vi "Main FPGA 8-axis with Limits and changes 16DIO.vi"() -> ()   [LabVIEW 2013]
uses:
  <vilib>/Motion/MotorControl/_s/nism.interpretControlRegister.stateTransition.ctl
  <vilib>/Platform/TimedLoop/XDataNode/timing_clust.ctl
  <vilib>/Platform/TimedLoop/XDataNode/nitl_modes.ctl
  <vilib>/Platform/TimedLoop/XDataNode/wakeup.ctl
  <vilib>/rvi/Emulation/niFpgaSctlEmulationGetInTimedLoop.vi
  <vilib>/rvi/Emulation/niFpgaEmulationReportErrorSimple.vi
  <vilib>/rvi/Emulation/niFpgaGetClockAttributes.vi
  <vilib>/rvi/Emulation/niFpgaCriticalErrorInLSC.vi
  Global FPGA 8-axis.vi
  <vilib>/rvi/eio/common/nirviEmuTemplateMethod_errors.vi
  <vilib>/Motion/SoftMotion/Synchronization/nism.rioScan.generateSyncScan.vi
  <vilib>/rvi/Emulation/niFpgaProcessEmulError.vi
  <vilib>/Motion/MotorControl/_s/nism.interpretControlRegister.indexed.vi
  <vilib>/Motion/MotorControl/_s/nism.generateStatusRegister.indexed.vi
  <vilib>/Motion/MotorControl/_s/nism.mdo.read.dio.portA.2.vi
  <vilib>/Motion/MotorControl/_s/nism.mdo.read.positionLoopSyncData.vi
  <vilib>/Motion/MotorControl/_s/nism.mdo.read.splineData.vi
  <vilib>/Motion/MotorControl/_s/nism.splineInterpolation.fxp.3.index.vi
  <vilib>/Motion/MotorControl/_s/nism.mdo.handler.indexed.vi
  <vilib>/Platform/TimedLoop/XDataNode/XDataNode.xnode
  <vilib>/eio/EIONode/EIONode.xnode
  <vilib>/Motion/MotorControl/NI_SoftMotion_MotorControlIP.lvlib
  <vilib>/Platform/TimedLoop/XDataNode/XDNodeRunTimeDep.lvlib
  <vilib>/Motion/SoftMotion/Synchronization/NI_SoftMotion_Synchronization.lvlib
panel:
  out "DI (8bits)":u8
  in  "DO (8bits)":u32
  out "Axis Positions":fxp<+/-,64,32>[](array[numeric])
  in  "STEP or CW? (T=STEP)":bool
  out "Drive Enable":bool[](array[boolean])
  in  "Enable Watchdog":bool
  in  "Pet Watchdog":bool
  in  "Watchdog Timeout Period (ticks)":u64=40000000 format="%.0p"
  out "Watchdog Timed Out?":bool
  out "Time Since Last Pet":u64
  in  "Enable value":bool
  in  "Drive Enable override?":bool
  out "State":T1=enum."Start --> Initializing" caption="state transition"
  in  "Sync Value":bool
  in  "Sync Enable override?":bool
  in  "Invert direction?":bool
  out "Sync is Fault":bool
  out "Sync is Locked":bool
  in  "minimum pulse":u16=40
  # "Synchronization Loop"
  # "Control Status Loop"
  # "Notes: \n1. This VI provides the communication interface between the NI SoftMotion Engine and the LabVIEW FPGA Module. You must compile this VI for a specific FPGA target before use. After compiling, run the VI before running any of the Express VI examples. For information on moving this example to another FPGA target, refer to ni.com/info and enter info code fpgaex.\n\n2. Only use the Reset Axis button if you are unable to communicate with the axis by any other means. This button resets the device state machine and other VIs to a known state. After resetting the axis, switch the NI Scan Engine from Active Mode to Configuration Mode, then back to Active Mode, before attempting to enable the axis."
  # "(These two buttons \nare for testing\npurposes.)"
  # "(These two buttons \nare for testing\npurposes.)"
  # "Step/Direction Loop"
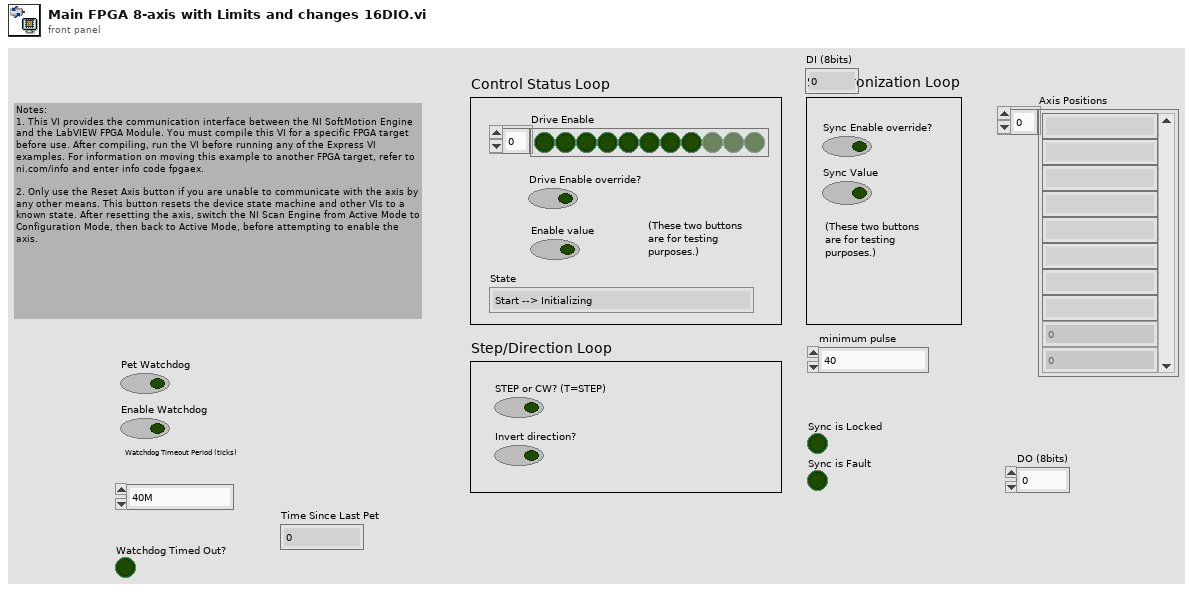
[diagram p1: front panel]
types:
  T1 = typedef "NI_SoftMotion_MotorControlIP.lvlib/nism.interpretControlRegister.stateTransition.ctl" = enum8{"Invalid", "Start --> Initializing", "Initializing --> Disabled", "Disabled --> Ready To Switch On", "Ready To Switch On --> Switched On", "Ready To Switch On --> Disable", "Switched On --> Operation Enable", "Switched On --> Ready To Switch On", "Switched On --> Disabled", "Operation Enable --> Switched On", "Operation Enable --> Ready To Switch On", "Operation Enable --> Disabled", "Fault --> Disabled", "Any --> Fault", "None"}
  T2 = typedef "NI_SoftMotion_MotorControlIP.lvlib/nism.dio.portA.config.2.ctl" = cluster{"digital filter (us)":u16[], "safe state":enum16{"Low", "High", "No Change"}[]}
  T3 = typedef "NI_SoftMotion_MotorControlIP.lvlib/nism.mdo.splineData.ctl" = cluster{"spline type":T4, "traj per/spline per":u16, "spline per/traj per":fxp<+,32,0>}
  T4 = typedef "nism.splineInterpolation.type.ctl" = u16
  T5 = typedef "NI_SoftMotion_Synchronization.lvlib/nism.softmotionScan.timerConfig.ctl" = cluster{"Target Period (clocks)":u16, "Host Period / Target Period":u16}
  T6 = typedef "NI_SoftMotion_Synchronization.lvlib/nism.softmotionScan.timerControl.ctl" = cluster{"SM Scan":bool, "SM Scan Count":u32, "SM Scan Enabled":bool}
  T7 = typedef "XDNodeRunTimeDep.lvlib/timing_clust.ctl" = cluster{"Expected End [f-1]":u64, "Actual End [f-1]":u64, "Finished Late? [f-1]":bool, "Expected End [i-1]":u64, "Actual End [i-1]":u64, "Finished Late? [i-1]":bool, "Expected Start [i]":u64, "Actual Start [i]":u64, "Expected Start [f]":u64, "Actual Start [f]":u64, "Source Name":string, "Structure Name":string, "Period":i64, "Deadline":i64, "Offset":i64, "Start":i64, "Priority":i32, "Timeout":i32, "Mode":T8, "Wakeup Reason":T9, "Error":errorcluster, "Source Type":string, "Secondary Source Type":string, "Global End Time":u64, "Global Start Time":u64, "Frame Duration":u64, "Iteration Duration":u64, "Assigned CPU":i32, "I/O Scan Engine Mode":u32}
  T8 = typedef "XDNodeRunTimeDep.lvlib/nitl_modes.ctl" = enum32{"No Change", "Process missed periods, maintain original phase", "Discard missed periods, maintain original phase", "Process missed periods, ignore original phase", "Discard missed periods, ignore original phase"}
  T9 = typedef "XDNodeRunTimeDep.lvlib/wakeup.ctl" = enum32{"Normal", "Aborted", "Asynchronous wakeup", "Timing source error", "Timed loop error", "Timeout"}
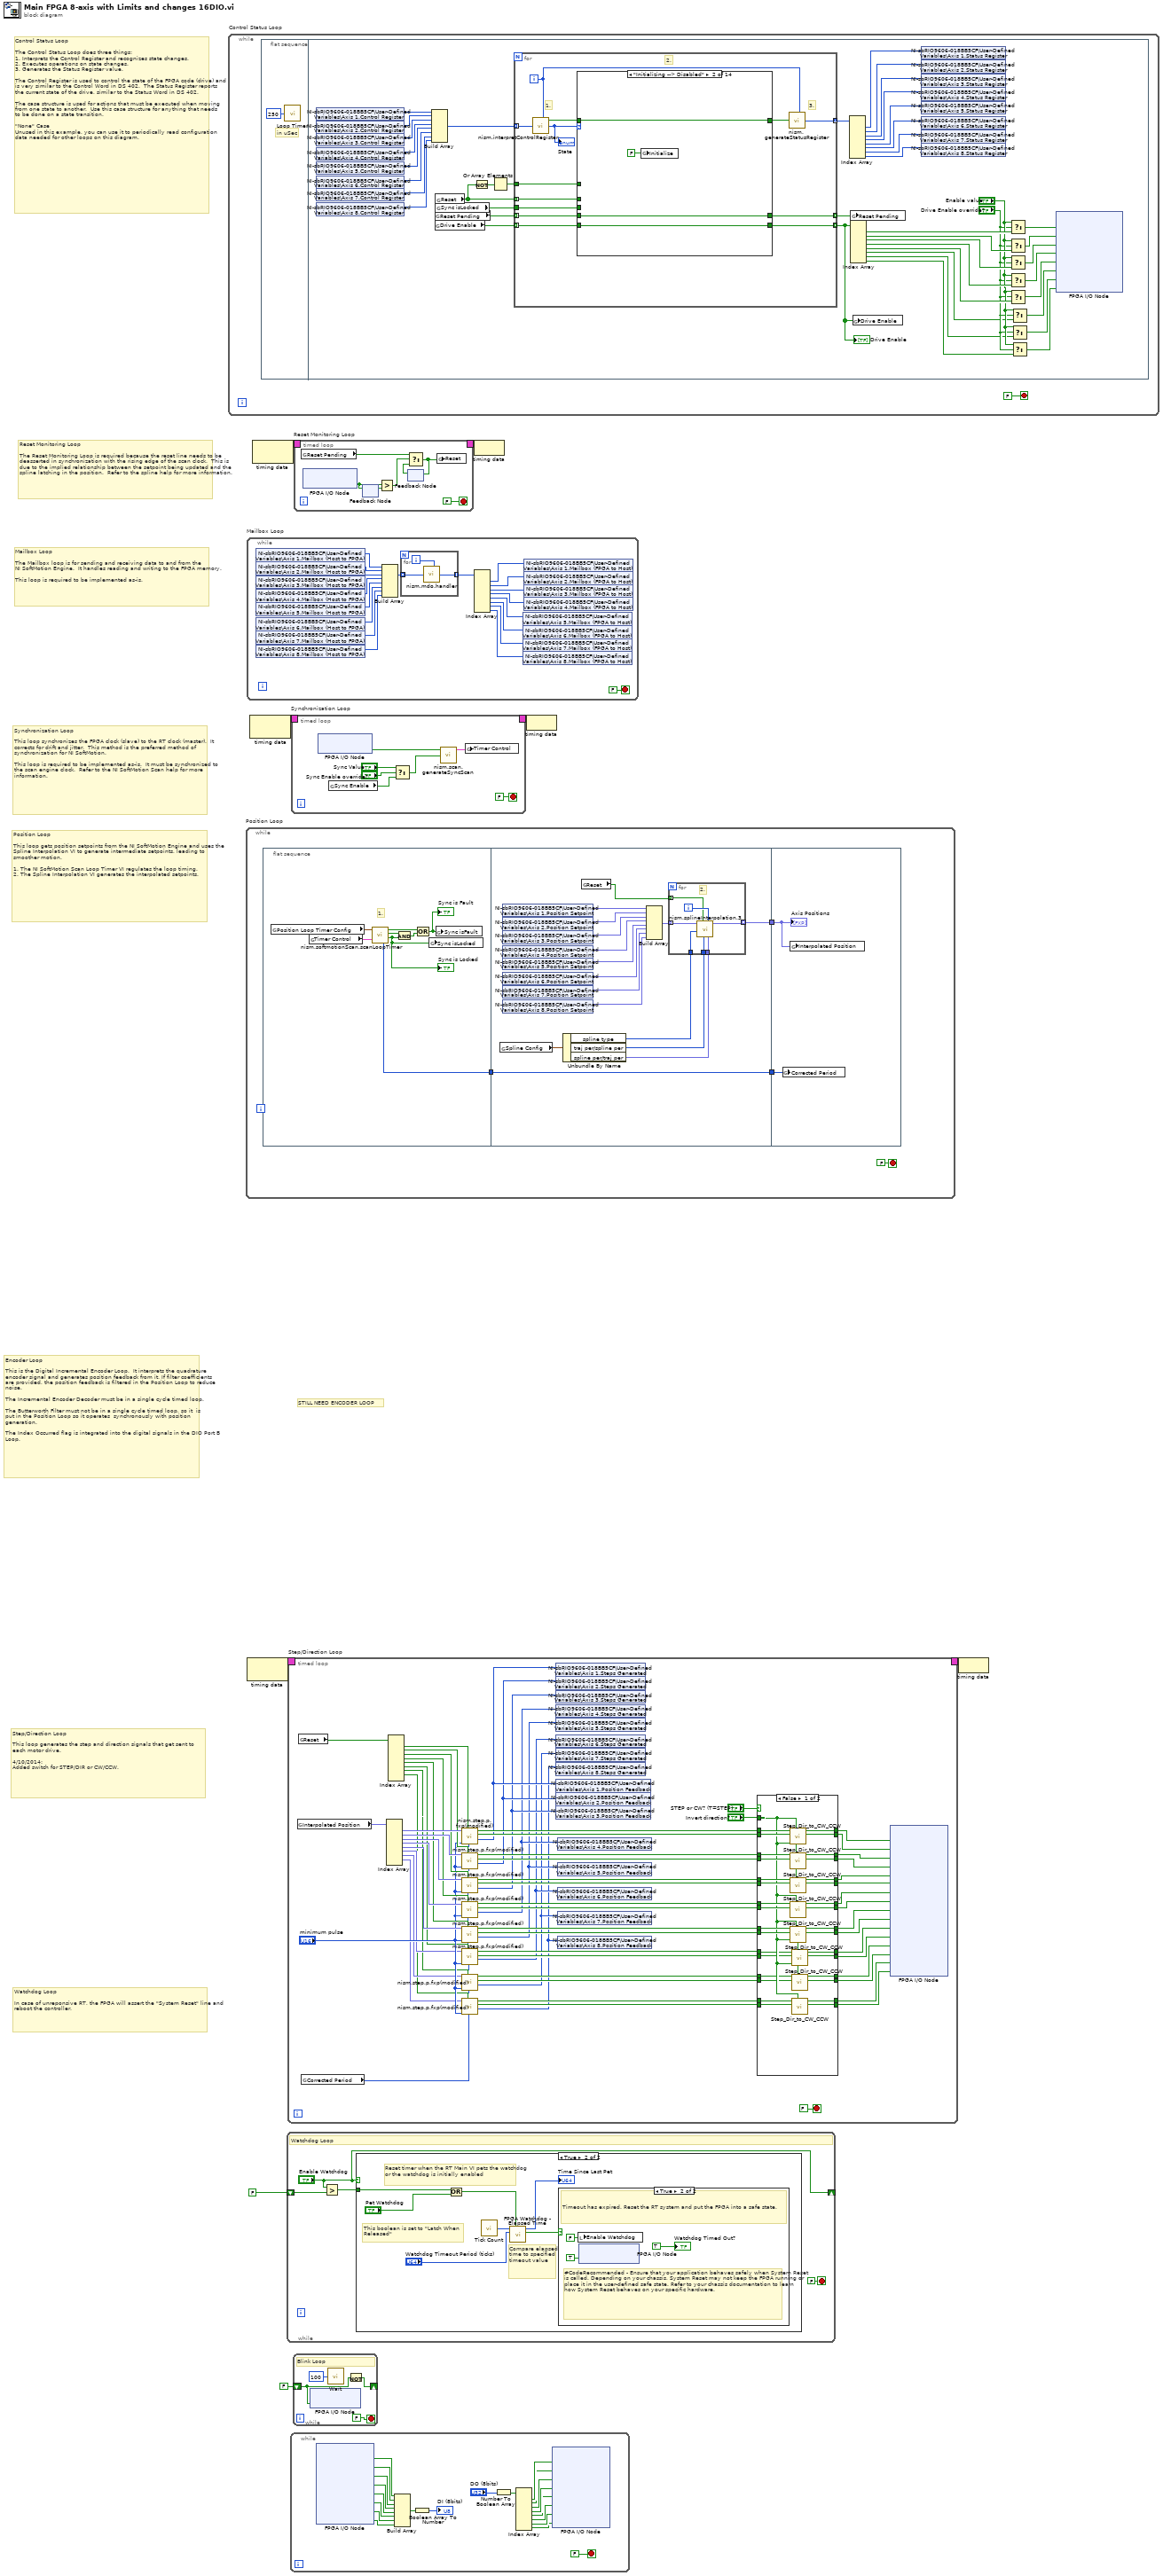
[diagram p0: block diagram]
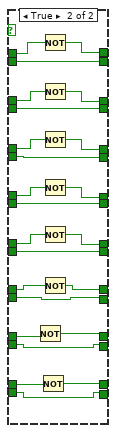
[diagram p5: hidden frame]
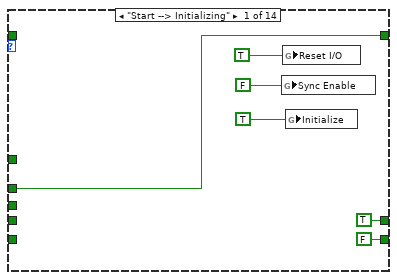
[diagram p6: hidden frame]
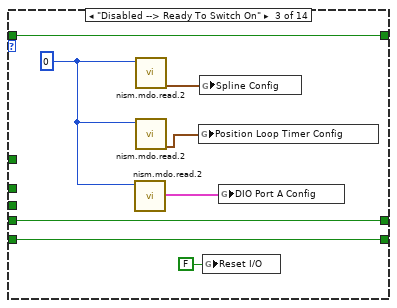
[diagram p7: hidden frame]
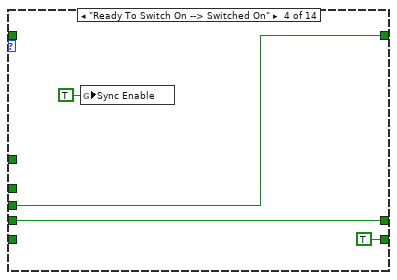
[diagram p8: hidden frame]
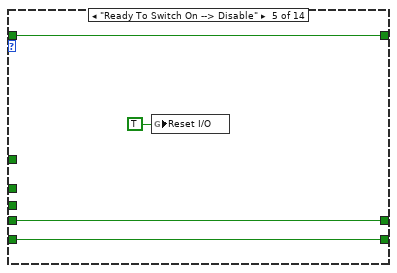
[diagram p9: hidden frame]
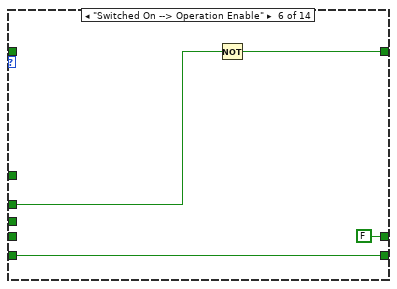
[diagram p10: hidden frame]
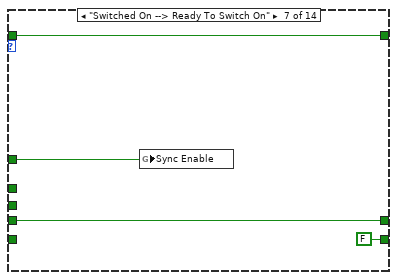
[diagram p11: hidden frame]
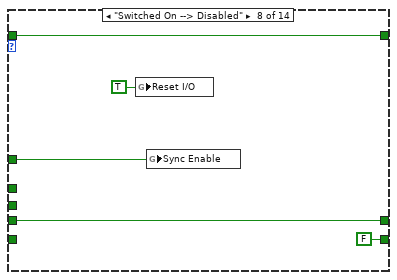
[diagram p12: hidden frame]
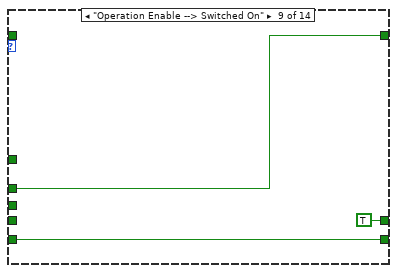
[diagram p13: hidden frame]
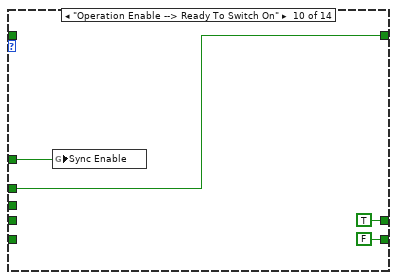
[diagram p14: hidden frame]
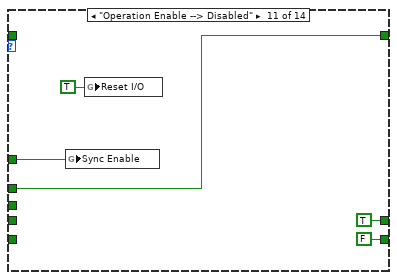
[diagram p15: hidden frame]
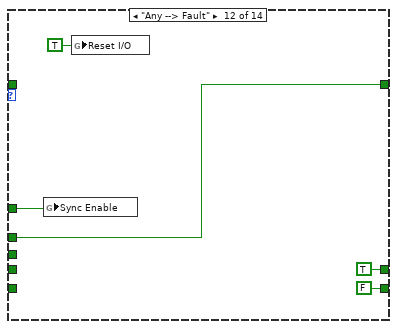
[diagram p16: hidden frame]
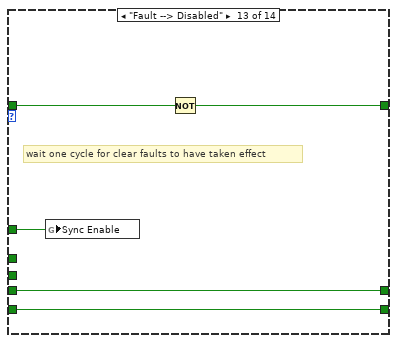
[diagram p17: hidden frame]
diagram:
  # "STILL NEED ENCODER LOOP"
  # "Encoder Loop\n\nThis is the Digital Incremental Encoder Loop.  It interprets the quadrature encoder signal and generates position feedback from it. If filter coefficients are provided, the position feedback is filtered in the Position Loop to reduce noise.\n\nThe Incremental Encoder Decoder must be in a single cycle timed loop.\n\nThe Butterworth Filter must not be in a single cycle timed loop, so it  is\nput in the Position Loop so it operates  synchronously with position generation.\n\nThe Index Occurred flag is integrated into the digital signals in the DIO Port B Loop."
  # "Watchdog Loop\n\nIn case of unreponsive RT, the FPGA will assert the \"System Reset\" line and reboot the controller."
  # "Step/Direction Loop\n\nThis loop generates the step and direction signals that get sent to \neach motor drive.\n\n4/10/2014:\nAdded switch for STEP/DIR or CW/CCW."
  # "Position Loop\n\nThis loop gets position setpoints from the NI SoftMotion Engine and uses the Spline Interpolation VI to generate intermediate setpoints, leading to smoother motion.\n\n1. The NI SoftMotion Scan Loop Timer VI regulates the loop timing. \n2. The Spline Interpolation VI generates the interpolated setpoints."
  # "Synchronization Loop\n\nThis loop synchronizes the FPGA clock (slave) to the RT clock (master).  It corrects for drift and jitter.  This method is the preferred method of synchronization for NI SoftMotion.\n\nThis loop is required to be implemented as-is.  It must be synchronized to the scan engine clock.  Refer to the NI SoftMotion Scan help for more information."
  # "Mailbox Loop\n\nThe Mailbox loop is for sending and receiving data to and from the \nNI SoftMotion Engine.  It handles reading and writing to the FPGA memory.\n\nThis loop is required to be implemented as-is."
  # "Reset Monitoring Loop\n\nThe Reset Monitoring Loop is required because the reset line needs to be deasserted in synchronization with the rising edge of the scan clock.  This is due to the implied relationship between the setpoint being updated and the spline latching in the position.  Refer to the spline help for more information."
  # "Control Status Loop\n\nThe Control Status Loop does three things:\n1. Interprets the Control Register and recognizes state changes.\n2. Executes operations on state changes.\n3. Generates the Status Register value.\n\nThe Control Register is used to control the state of the FPGA code (drive) and is very similar to the Control Word in DS 402.  The Status Register reports the current state of the drive, similar to the Status Word in DS 402.\n\nThe case structure is used for actions that must be executed when moving from one state to another.  Use this case structure for anything that needs to be done on a state transition.\n\n\"None\" Case\nUnused in this example, you can use it to periodically read configuration data needed for other loops on this diagram."
  n1 = while "Control Status Loop" {
    stop <- FALSE stop-if-true
    n2 = flat-sequence {
      frame #0 {
        # "in uSec"
        n3 = call "Loop Timer"("Count(uSec)"=u32 250) -> ()  [unwired: 1 out]
      }
      frame #1 {
        n4 = shared-variable "NI-sbRIO9606-018BB5CF\\User-Defined Variables\\Axis 1.Control Register"() -> (w44:u32)  [unwired: 1 in, 1 out]
        n5 = shared-variable "NI-sbRIO9606-018BB5CF\\User-Defined Variables\\Axis 2.Control Register"() -> (w43:u32)  [unwired: 1 in, 1 out]
        n6 = shared-variable "NI-sbRIO9606-018BB5CF\\User-Defined Variables\\Axis 3.Control Register"() -> (w42:u32)  [unwired: 1 in, 1 out]
        n7 = shared-variable "NI-sbRIO9606-018BB5CF\\User-Defined Variables\\Axis 4.Control Register"() -> (w41:u32)  [unwired: 1 in, 1 out]
        n8 = shared-variable "NI-sbRIO9606-018BB5CF\\User-Defined Variables\\Axis 5.Control Register"() -> (w40:u32)  [unwired: 1 in, 1 out]
        n9 = shared-variable "NI-sbRIO9606-018BB5CF\\User-Defined Variables\\Axis 6.Control Register"() -> (w24:u32)  [unwired: 1 in, 1 out]
        n10 = shared-variable "NI-sbRIO9606-018BB5CF\\User-Defined Variables\\Axis 7.Control Register"() -> (w23:u32)  [unwired: 1 in, 1 out]
        n11 = shared-variable "NI-sbRIO9606-018BB5CF\\User-Defined Variables\\Axis 8.Control Register"() -> (w22:u32)  [unwired: 1 in, 1 out]
        n12 = Build Array(w44, w43, w42, w41, w40, w24, w23, w22) -> (w53:u32[])
        n13 = global read "Global FPGA 8-axis.vi" "Reset Pending"() -> (w48:bool[])
        n14 = global read "Global FPGA 8-axis.vi" "Drive Enable"() -> (w47:bool[])
        n15 = global read "Global FPGA 8-axis.vi" "Reset"() -> (w49:bool[])
        n16 = global read "Global FPGA 8-axis.vi" "Sync isLocked"() -> (w54:bool)
        n17 = Not(x=w49) -> (.not. x?=w51:bool[])
        n18 = Or Array Elements(Boolean array=w51) -> (logical OR=w50:bool)
        n19 = for {
          tunnel: w49 -> [w62] mode=indexing
          tunnel: w54 -> [w61]
          tunnel: w53 -> [w63] mode=indexing
          tunnel: [w60] -> w45 mode=indexing
          tunnel: [w59] -> w52 mode=indexing
          tunnel: [w58] -> w46 mode=indexing
          tunnel: w50 -> [w57]
          tunnel: w48 -> [w56] mode=indexing
          tunnel: w47 -> [w55] mode=indexing
          i -> [w64]
          # "3."
          # "2."
          # "1."
          n20 = call-poly <vilib>:"nism.interpretControlRegister.vi"("control register"=w63, "axis index"=w64) -> ("transition occurred"=w65:bool, "state transition"=w66:T1)  [unwired: 6 in]
          "State" <- w66
          n21 = case shown="\"Initializing --> Disabled\"" w66 {
            tunnel: w65 -> [_ w77 w85 _ w93 _ w101 w106 _ _ _ _ w128 _]
            tunnel: [w73 w77 w85 w87 w93 w97 w101 w106 w108 w111 w116 w121 w127 _] -> w67
            tunnel: w62 -> [w73 _ _ _ _ w96 _ _ w108 w111 w116 w121 _ _]
            tunnel: w61 -> [_ _ _ w87 _ _ _ _ _ _ _ _ _ _]
            tunnel: [TRUE ("Write.Reset Pending") w76 w82 w86 w92 FALSE ("Write.Reset Pending") w98 w103 TRUE ("Write.Reset Pending") TRUE ("Write.Reset Pending") TRUE ("Write.Reset Pending") TRUE ("Write.Reset Pending") w125 w130] -> w59
            tunnel: [FALSE ("Write.Drive Enable") w75 w81 TRUE ("Write.Drive Enable") w91 w94 FALSE ("Write.Drive Enable") FALSE ("Write.Drive Enable") w107 FALSE ("Write.Drive Enable") FALSE ("Write.Drive Enable") FALSE ("Write.Drive Enable") w124 w129] -> w58
            tunnel: w57 -> [_ _ _ _ _ _ w99 w104 _ w110 w115 w120 w126 _]
            tunnel: w56 -> [_ w76 w82 w86 w92 _ w98 w103 _ _ _ _ w125 w130]
            tunnel: w55 -> [_ w75 w81 _ w91 w94 _ _ w107 _ _ _ w124 w129]
            frame "Start --> Initializing" {
              n22 = global write "Global FPGA 8-axis.vi" "Sync Enable"(FALSE ("Sync Enable")) -> ()
              n23 = global write "Global FPGA 8-axis.vi" "Reset I/O"(TRUE ("Reset I/O")) -> ()
              n24 = global write "Global FPGA 8-axis.vi" "Initialize"(TRUE ("Reset I/O")) -> ()
            }
            frame "Initializing --> Disabled" {
              n25 = global write "Global FPGA 8-axis.vi" "Initialize"(FALSE ("Reset I/O")) -> ()
            }
            frame "Disabled --> Ready To Switch On" {
              w79 = 0 ("axis index")
              n26 = call-poly <vilib>:"nism.mdo.read.2.vi"("axis index"=w79) -> ("dio config (port a)"=w78:T2)  [unwired: 10 in]
              n27 = call-poly <vilib>:"nism.mdo.read.2.vi"("axis index"=w79) -> ("spline"=w84:T3)  [unwired: 10 in]
              n28 = call-poly <vilib>:"nism.mdo.read.2.vi"("axis index"=w79) -> ("position loop sync"=w83:T5)  [unwired: 10 in]
              n29 = global write "Global FPGA 8-axis.vi" "Position Loop Timer Config"(w83) -> ()
              n30 = global write "Global FPGA 8-axis.vi" "Spline Config"(w84) -> ()
              n31 = global write "Global FPGA 8-axis.vi" "Reset I/O"(FALSE ("Reset I/O")) -> ()
              n32 = global write "Global FPGA 8-axis.vi" "DIO Port A Config"(w78) -> ()
            }
            frame "Ready To Switch On --> Switched On" {
              n33 = global write "Global FPGA 8-axis.vi" "Sync Enable"(TRUE ("Sync Enable")) -> ()
            }
            frame "Ready To Switch On --> Disable" {
              n34 = global write "Global FPGA 8-axis.vi" "Reset I/O"(TRUE ("Reset I/O")) -> ()
            }
            frame "Switched On --> Operation Enable" {
              n35 = Not(x=w96) -> (.not. x?=w97:bool)
            }
            frame "Switched On --> Ready To Switch On" {
              n36 = global write "Global FPGA 8-axis.vi" "Sync Enable"(w99) -> ()
            }
            frame "Switched On --> Disabled" {
              n37 = global write "Global FPGA 8-axis.vi" "Reset I/O"(TRUE ("Reset I/O")) -> ()
              n38 = global write "Global FPGA 8-axis.vi" "Sync Enable"(w104) -> ()
            }
            frame "Operation Enable --> Switched On" {
            }
            frame "Operation Enable --> Ready To Switch On" {
              n39 = global write "Global FPGA 8-axis.vi" "Sync Enable"(w110) -> ()
            }
            frame "Operation Enable --> Disabled" {
              n40 = global write "Global FPGA 8-axis.vi" "Sync Enable"(w115) -> ()
              n41 = global write "Global FPGA 8-axis.vi" "Reset I/O"(TRUE ("Reset I/O")) -> ()
            }
            frame "Any --> Fault" {
              n42 = global write "Global FPGA 8-axis.vi" "Sync Enable"(w120) -> ()
              n43 = global write "Global FPGA 8-axis.vi" "Reset I/O"(TRUE ("Reset I/O")) -> ()
            }
            frame "Fault --> Disabled" {
              # "wait one cycle for clear faults to have taken effect"
              n44 = global write "Global FPGA 8-axis.vi" "Sync Enable"(w126) -> ()
              n45 = Not(x=w128) -> (.not. x?=w127:bool)
            }
            frame "None", Default {
            }
          }
          n46 = call-poly <vilib>:"nism.generateStatusRegister.vi"("transition success"=w67, "axis index"=w64) -> ("status register"=w60:u32)  [unwired: 7 in]
        }
        "Drive Enable" <- w46
        n47 = Index Array(array=w45) -> (element #1=w39:u32, element #2=w38:u32, element #3=w37:u32, element #4=w36:u32, element #5=w35:u32, element #6=w21:u32, element #7=w20:u32, element #8=w19:u32)  [unwired: 8 in]
        n48 = global write "Global FPGA 8-axis.vi" "Reset Pending"(w52) -> ()
        n49 = Index Array(array=w46) -> (element #1=w34:bool, element #2=w32:bool, element #3=w30:bool, element #4=w28:bool, element #5=w26:bool, element #6=w16:bool, element #7=w15:bool, element #8=w14:bool)  [unwired: 8 in]
        n50 = global write "Global FPGA 8-axis.vi" "Drive Enable"(w46) -> ()
        n51 = shared-variable "NI-sbRIO9606-018BB5CF\\User-Defined Variables\\Axis 1.Status Register"(w39) -> ()  [unwired: 1 in, 1 out]
        n52 = shared-variable "NI-sbRIO9606-018BB5CF\\User-Defined Variables\\Axis 2.Status Register"(w38) -> ()  [unwired: 1 in, 1 out]
        n53 = shared-variable "NI-sbRIO9606-018BB5CF\\User-Defined Variables\\Axis 3.Status Register"(w37) -> ()  [unwired: 1 in, 1 out]
        n54 = shared-variable "NI-sbRIO9606-018BB5CF\\User-Defined Variables\\Axis 4.Status Register"(w36) -> ()  [unwired: 1 in, 1 out]
        n55 = shared-variable "NI-sbRIO9606-018BB5CF\\User-Defined Variables\\Axis 5.Status Register"(w35) -> ()  [unwired: 1 in, 1 out]
        n56 = shared-variable "NI-sbRIO9606-018BB5CF\\User-Defined Variables\\Axis 6.Status Register"(w21) -> ()  [unwired: 1 in, 1 out]
        n57 = shared-variable "NI-sbRIO9606-018BB5CF\\User-Defined Variables\\Axis 7.Status Register"(w20) -> ()  [unwired: 1 in, 1 out]
        n58 = shared-variable "NI-sbRIO9606-018BB5CF\\User-Defined Variables\\Axis 8.Status Register"(w19) -> ()  [unwired: 1 in, 1 out]
        n59 = Select(t="Enable value", s="Drive Enable override?", f=w34) -> (s? t:f=w33:bool)
        n60 = Select(t="Enable value", s="Drive Enable override?", f=w32) -> (s? t:f=w31:bool)
        n61 = Select(t="Enable value", s="Drive Enable override?", f=w30) -> (s? t:f=w29:bool)
        n62 = Select(t="Enable value", s="Drive Enable override?", f=w28) -> (s? t:f=w27:bool)
        n63 = Select(t="Enable value", s="Drive Enable override?", f=w26) -> (s? t:f=w25:bool)
        n64 = Select(t="Enable value", s="Drive Enable override?", f=w16) -> (s? t:f=w13:bool)
        n65 = Select(t="Enable value", s="Drive Enable override?", f=w15) -> (s? t:f=w12:bool)
        n66 = Select(t="Enable value", s="Drive Enable override?", f=w14) -> (s? t:f=w11:bool)
        n67 = xnode "FPGA I/O Node"("Axis1_Servo On"=w33, "Axis2_Servo On"=w31, "Axis3_Servo On"=w29, "Axis4_Servo On"=w27, "Axis5_Servo On"=w25, "RMC/DIO1"=w13, "RMC/DIO2"=w12, "RMC/DIO3"=w11) -> ()  [unwired: 8 in, 8 out]
      }
    }
  }
  n68 = while "Position Loop" {
    stop <- FALSE stop-if-true
    n69 = flat-sequence {
      tunnel: [w135] -> w131
      tunnel: [w152] -> w133
      tunnel: [w151] -> w132
      tunnel: w131 -> [w151]
      tunnel: w133 -> [w166]
      tunnel: w132 -> [w167]
      frame #0 {
        # "1."
        n70 = global read "Global FPGA 8-axis.vi" "Position Loop Timer Config"() -> (w137:T5)
        n71 = global read "Global FPGA 8-axis.vi" "Timer Control"() -> (w136:T6)
        n72 = call <vilib>:"nism.softmotionScan.scanLoopTimer.vi"("Timer Control"=w136, "Timer Config"=w137) -> ("Scan Running?"=w139:bool, "Finished Late?"=w141:bool, "Fault Occurred?"=w142:bool, "Corrected Period"=w135:u16)  [unwired: 5 in, 1 out]
        "Sync is Locked" <- w139
        n73 = Compound Arithmetic op=AND(w141, w139) -> (w140:bool)
        n74 = Compound Arithmetic op=OR(w142, w140) -> (w138:bool)
        "Sync is Fault" <- w138
        n75 = global write "Global FPGA 8-axis.vi" "Sync isLocked"(w139) -> ()
        n76 = global write "Global FPGA 8-axis.vi" "Sync isFault"(w138) -> ()
      }
      frame #1 {
        n77 = global read "Global FPGA 8-axis.vi" "Spline Config"() -> (w154:T3)
        n78 = shared-variable "NI-sbRIO9606-018BB5CF\\User-Defined Variables\\Axis 1.Position Setpoint"() -> (w150:fxp<+/-,64,32>)  [unwired: 1 in, 1 out]
        n79 = shared-variable "NI-sbRIO9606-018BB5CF\\User-Defined Variables\\Axis 2.Position Setpoint"() -> (w149:fxp<+/-,64,32>)  [unwired: 1 in, 1 out]
        n80 = shared-variable "NI-sbRIO9606-018BB5CF\\User-Defined Variables\\Axis 3.Position Setpoint"() -> (w148:fxp<+/-,64,32>)  [unwired: 1 in, 1 out]
        n81 = shared-variable "NI-sbRIO9606-018BB5CF\\User-Defined Variables\\Axis 4.Position Setpoint"() -> (w147:fxp<+/-,64,32>)  [unwired: 1 in, 1 out]
        n82 = shared-variable "NI-sbRIO9606-018BB5CF\\User-Defined Variables\\Axis 5.Position Setpoint"() -> (w146:fxp<+/-,64,32>)  [unwired: 1 in, 1 out]
        n83 = shared-variable "NI-sbRIO9606-018BB5CF\\User-Defined Variables\\Axis 6.Position Setpoint"() -> (w145:fxp<+/-,64,32>)  [unwired: 1 in, 1 out]
        n84 = shared-variable "NI-sbRIO9606-018BB5CF\\User-Defined Variables\\Axis 7.Position Setpoint"() -> (w144:fxp<+/-,64,32>)  [unwired: 1 in, 1 out]
        n85 = shared-variable "NI-sbRIO9606-018BB5CF\\User-Defined Variables\\Axis 8.Position Setpoint"() -> (w143:fxp<+/-,64,32>)  [unwired: 1 in, 1 out]
        n86 = Unbundle By Name(w154) -> ("spline type"=w158:T4, "traj per/spline per"=w157:u16, "spline per/traj per"=w156:fxp<+,32,0>)
        n87 = global read "Global FPGA 8-axis.vi" "Reset"() -> (w153:bool[])
        n88 = Build Array(w150, w149, w148, w147, w146, w145, w144, w143) -> (w155:fxp<+/-,64,32>[])
        n89 = for {
          tunnel: w158 -> [w165]
          tunnel: w157 -> [w164]
          tunnel: w156 -> [w163]
          tunnel: w153 -> [w160] mode=indexing
          tunnel: w155 -> [w162] mode=indexing
          tunnel: [w159] -> w152 mode=indexing
          i -> [w161]
          # "2."
          n90 = call-poly <vilib>:"nism.splineInterpolation.3.vi"("1 / calls per sample"=w163, "index"=w161, "calls per sample"=w164, "reset"=w160, "spline type"=w165, "x"=w162) -> ("xi"=w159:fxp<+/-,64,32>)  [unwired: 5 in]
        }
      }
      frame #2 {
        n91 = global write "Global FPGA 8-axis.vi" "Corrected Period"(w167) -> ()
        n92 = global write "Global FPGA 8-axis.vi" "Interpolated Position"(w166) -> ()
        "Axis Positions" <- w166
      }
    }
  }
  n93 = while "Mailbox Loop" {
    stop <- FALSE stop-if-true
    n94 = shared-variable "NI-sbRIO9606-018BB5CF\\User-Defined Variables\\Axis 1.Mailbox (Host to FPGA)"() -> (w183:u64)  [unwired: 1 in, 1 out]
    n95 = shared-variable "NI-sbRIO9606-018BB5CF\\User-Defined Variables\\Axis 2.Mailbox (Host to FPGA)"() -> (w182:u64)  [unwired: 1 in, 1 out]
    n96 = shared-variable "NI-sbRIO9606-018BB5CF\\User-Defined Variables\\Axis 3.Mailbox (Host to FPGA)"() -> (w181:u64)  [unwired: 1 in, 1 out]
    n97 = shared-variable "NI-sbRIO9606-018BB5CF\\User-Defined Variables\\Axis 4.Mailbox (Host to FPGA)"() -> (w180:u64)  [unwired: 1 in, 1 out]
    n98 = shared-variable "NI-sbRIO9606-018BB5CF\\User-Defined Variables\\Axis 5.Mailbox (Host to FPGA)"() -> (w179:u64)  [unwired: 1 in, 1 out]
    n99 = shared-variable "NI-sbRIO9606-018BB5CF\\User-Defined Variables\\Axis 6.Mailbox (Host to FPGA)"() -> (w173:u64)  [unwired: 1 in, 1 out]
    n100 = shared-variable "NI-sbRIO9606-018BB5CF\\User-Defined Variables\\Axis 7.Mailbox (Host to FPGA)"() -> (w172:u64)  [unwired: 1 in, 1 out]
    n101 = shared-variable "NI-sbRIO9606-018BB5CF\\User-Defined Variables\\Axis 8.Mailbox (Host to FPGA)"() -> (w171:u64)  [unwired: 1 in, 1 out]
    n102 = Build Array(w183, w182, w181, w180, w179, w173, w172, w171) -> (w185:u64[])
    n103 = for {
      tunnel: w185 -> [w189] mode=indexing
      tunnel: [w188] -> w184 mode=indexing
      i -> [w187]
      n104 = call-poly <vilib>:"nism.mdo.handler.vi"("mbox (host to fpga)"=w189, "axis index"=w187) -> ("mbox (fpga to host)"=w188:u64)  [unwired: 7 in]
    }
    n105 = Index Array(array=w184) -> (element #1=w178:u64, element #2=w177:u64, element #3=w176:u64, element #4=w175:u64, element #5=w174:u64, element #6=w170:u64, element #7=w169:u64, element #8=w168:u64)  [unwired: 8 in]
    n106 = shared-variable "NI-sbRIO9606-018BB5CF\\User-Defined Variables\\Axis 6.Mailbox (FPGA to Host)"(w170) -> ()  [unwired: 1 in, 1 out]
    n107 = shared-variable "NI-sbRIO9606-018BB5CF\\User-Defined Variables\\Axis 7.Mailbox (FPGA to Host)"(w169) -> ()  [unwired: 1 in, 1 out]
    n108 = shared-variable "NI-sbRIO9606-018BB5CF\\User-Defined Variables\\Axis 8.Mailbox (FPGA to Host)"(w168) -> ()  [unwired: 1 in, 1 out]
    n109 = shared-variable "NI-sbRIO9606-018BB5CF\\User-Defined Variables\\Axis 5.Mailbox (FPGA to Host)"(w174) -> ()  [unwired: 1 in, 1 out]
    n110 = shared-variable "NI-sbRIO9606-018BB5CF\\User-Defined Variables\\Axis 1.Mailbox (FPGA to Host)"(w178) -> ()  [unwired: 1 in, 1 out]
    n111 = shared-variable "NI-sbRIO9606-018BB5CF\\User-Defined Variables\\Axis 2.Mailbox (FPGA to Host)"(w177) -> ()  [unwired: 1 in, 1 out]
    n112 = shared-variable "NI-sbRIO9606-018BB5CF\\User-Defined Variables\\Axis 3.Mailbox (FPGA to Host)"(w176) -> ()  [unwired: 1 in, 1 out]
    n113 = shared-variable "NI-sbRIO9606-018BB5CF\\User-Defined Variables\\Axis 4.Mailbox (FPGA to Host)"(w175) -> ()  [unwired: 1 in, 1 out]
  }
  n114 = node-c288() -> (w8:T7)  [unwired: 1 in]
  n115 = node-c288() -> (w6:T7)  [unwired: 1 in]
  n116 = node-c288() -> (w4:T7)  [unwired: 1 in]
  n117 = while "RT Watchdog Loop" {
    shift-right: ["Enable Watchdog"] -> _
    shift-left: FALSE ("Enable RT Watchdog") -> [w193]
    stop <- FALSE stop-if-true
    # "Watchdog Loop"
    n118 = Greater?(x="Enable Watchdog", y=w193) -> (0:w190:bool)
    n119 = case shown="True" "Enable Watchdog" {
      tunnel: w190 -> [_ w196]
      frame False {
        # "This loop has to be explicitly enabled from the RT Main VI.  This reduces the possiblity of an endless reboot cycle."
      }
      frame True {
        # "This boolean is set to \"Latch When Released\""
        # "Compare elapsed time to specified timeout value"
        # "Reset timer when the RT Main VI pets the watchdog or the watchdog is initially enabled"
        n120 = Or(x=w196, y="Pet Watchdog") -> (x .or. y?=w195:bool)
        n121 = call "Tick Count"() -> ("Tick Count(Ticks)"=w199:u32)
        n122 = call "FPGA Watchdog - Elapsed Time.vi"("Reset"=w195, "Timeout Period"="Watchdog Timeout Period (ticks)", "Current Time"=w199) -> ("Timeout"=w194:bool, "Elapsed Time"=→"Time Since Last Pet":u64)  [unwired: 7 in]
        n123 = case shown="True" w194 {
          frame False {
            # "Timeout has not expired."
          }
          frame True {
            # "#CodeRecommended - Ensure that your application behaves safely when System Reset is called. Depending on your chassis, System Reset may not keep the FPGA running or place it in the user-defined safe state. Refer to your chassis documentation to learn how System Reset behaves on your specific hardware."
            # "Timeout has expired. Reset the RT system and put the FPGA into a safe state."
            n124 = local write "Enable Watchdog"(FALSE ("Enable RT Watchdog")) -> ()
            n125 = xnode "FPGA I/O Node"("System Reset"=TRUE ("RT Reset on Watchdog Failure?")) -> ()  [unwired: 1 in, 1 out]
            "Watchdog Timed Out?" <- TRUE ("Watchdog Timed Out?")
          }
        }
      }
    }
  }
  n126 = timed-loop "Step/Direction Loop" {
    timing: w8 -> [_]
    timing-out: [_] -> w7
    stop <- FALSE stop-if-true
    n127 = global read "Global FPGA 8-axis.vi" "Interpolated Position"() -> (w265:fxp<+/-,64,32>[])
    n128 = global read "Global FPGA 8-axis.vi" "Reset"() -> (w259:bool[])
    n129 = global read "Global FPGA 8-axis.vi" "Corrected Period"() -> (w212:u16)
    n130 = Index Array(array=w265) -> (element #1=w264:fxp<+/-,64,32>, element #2=w263:fxp<+/-,64,32>, element #3=w262:fxp<+/-,64,32>, element #4=w261:fxp<+/-,64,32>, element #5=w260:fxp<+/-,64,32>, element #6=w224:fxp<+/-,64,32>, element #7=w223:fxp<+/-,64,32>, element #8=w222:fxp<+/-,64,32>)  [unwired: 9 in, 1 out]
    n131 = Index Array(array=w259) -> (element #1=w258:bool, element #2=w257:bool, element #3=w256:bool, element #4=w255:bool, element #5=w254:bool, element #6=w221:bool, element #7=w220:bool, element #8=w219:bool)  [unwired: 9 in, 1 out]
    n132 = call "nism.step.p.fxp(modified).vi"("calls per sample"=w212, "reset"=w258, "minimum pulse"="minimum pulse", "position setpoint"=w264) -> ("steps generated"=w211:i32, "step"=w252:bool, "direction"=w253:bool)  [unwired: 4 in, 1 out]
    n133 = call "nism.step.p.fxp(modified).vi"("calls per sample"=w212, "reset"=w257, "minimum pulse"="minimum pulse", "position setpoint"=w263) -> ("steps generated"=w210:i32, "step"=w250:bool, "direction"=w251:bool)  [unwired: 4 in, 1 out]
    n134 = call "nism.step.p.fxp(modified).vi"("calls per sample"=w212, "reset"=w256, "minimum pulse"="minimum pulse", "position setpoint"=w262) -> ("steps generated"=w209:i32, "step"=w248:bool, "direction"=w249:bool)  [unwired: 4 in, 1 out]
    n135 = call "nism.step.p.fxp(modified).vi"("calls per sample"=w212, "reset"=w255, "minimum pulse"="minimum pulse", "position setpoint"=w261) -> ("steps generated"=w208:i32, "step"=w246:bool, "direction"=w247:bool)  [unwired: 4 in, 1 out]
    n136 = call "nism.step.p.fxp(modified).vi"("calls per sample"=w212, "reset"=w254, "minimum pulse"="minimum pulse", "position setpoint"=w260) -> ("steps generated"=w207:i32, "step"=w244:bool, "direction"=w245:bool)  [unwired: 4 in, 1 out]
    n137 = call "nism.step.p.fxp(modified).vi"("calls per sample"=w212, "reset"=w221, "minimum pulse"="minimum pulse", "position setpoint"=w224) -> ("steps generated"=w206:i32, "step"=w230:bool, "direction"=w231:bool)  [unwired: 4 in, 1 out]
    n138 = call "nism.step.p.fxp(modified).vi"("calls per sample"=w212, "reset"=w220, "minimum pulse"="minimum pulse", "position setpoint"=w223) -> ("steps generated"=w205:i32, "step"=w228:bool, "direction"=w229:bool)  [unwired: 4 in, 1 out]
    n139 = call "nism.step.p.fxp(modified).vi"("calls per sample"=w212, "reset"=w219, "minimum pulse"="minimum pulse", "position setpoint"=w222) -> ("steps generated"=w204:i32, "step"=w226:bool, "direction"=w227:bool)  [unwired: 4 in, 1 out]
    n140 = shared-variable "NI-sbRIO9606-018BB5CF\\User-Defined Variables\\Axis 1.Steps Generated"(w211) -> ()  [unwired: 1 in, 1 out]
    n141 = shared-variable "NI-sbRIO9606-018BB5CF\\User-Defined Variables\\Axis 2.Steps Generated"(w210) -> ()  [unwired: 1 in, 1 out]
    n142 = shared-variable "NI-sbRIO9606-018BB5CF\\User-Defined Variables\\Axis 3.Steps Generated"(w209) -> ()  [unwired: 1 in, 1 out]
    n143 = shared-variable "NI-sbRIO9606-018BB5CF\\User-Defined Variables\\Axis 4.Steps Generated"(w208) -> ()  [unwired: 1 in, 1 out]
    n144 = shared-variable "NI-sbRIO9606-018BB5CF\\User-Defined Variables\\Axis 5.Steps Generated"(w207) -> ()  [unwired: 1 in, 1 out]
    n145 = shared-variable "NI-sbRIO9606-018BB5CF\\User-Defined Variables\\Axis 6.Steps Generated"(w206) -> ()  [unwired: 1 in, 1 out]
    n146 = shared-variable "NI-sbRIO9606-018BB5CF\\User-Defined Variables\\Axis 7.Steps Generated"(w205) -> ()  [unwired: 1 in, 1 out]
    n147 = shared-variable "NI-sbRIO9606-018BB5CF\\User-Defined Variables\\Axis 8.Steps Generated"(w204) -> ()  [unwired: 1 in, 1 out]
    n148 = shared-variable "NI-sbRIO9606-018BB5CF\\User-Defined Variables\\Axis 1.Position Feedback"(w211) -> ()  [unwired: 1 in, 1 out]
    n149 = shared-variable "NI-sbRIO9606-018BB5CF\\User-Defined Variables\\Axis 2.Position Feedback"(w210) -> ()  [unwired: 1 in, 1 out]
    n150 = shared-variable "NI-sbRIO9606-018BB5CF\\User-Defined Variables\\Axis 3.Position Feedback"(w209) -> ()  [unwired: 1 in, 1 out]
    n151 = shared-variable "NI-sbRIO9606-018BB5CF\\User-Defined Variables\\Axis 4.Position Feedback"(w208) -> ()  [unwired: 1 in, 1 out]
    n152 = shared-variable "NI-sbRIO9606-018BB5CF\\User-Defined Variables\\Axis 5.Position Feedback"(w207) -> ()  [unwired: 1 in, 1 out]
    n153 = shared-variable "NI-sbRIO9606-018BB5CF\\User-Defined Variables\\Axis 6.Position Feedback"(w206) -> ()  [unwired: 1 in, 1 out]
    n154 = shared-variable "NI-sbRIO9606-018BB5CF\\User-Defined Variables\\Axis 7.Position Feedback"(w205) -> ()  [unwired: 1 in, 1 out]
    n155 = shared-variable "NI-sbRIO9606-018BB5CF\\User-Defined Variables\\Axis 8.Position Feedback"(w204) -> ()  [unwired: 1 in, 1 out]
    n156 = case shown="False" "STEP or CW? (T=STEP)" {
      tunnel: w253 -> [w299 w331]
      tunnel: w252 -> [w298 w321]
      tunnel: w251 -> [w297 w329]
      tunnel: w250 -> [w296 w319]
      tunnel: w249 -> [w295 w327]
      tunnel: w248 -> [w294 w317]
      tunnel: w247 -> [w293 w325]
      tunnel: w246 -> [w292 w315]
      tunnel: w245 -> [w291 w323]
      tunnel: w244 -> [w290 w313]
      tunnel: "Invert direction?" -> [w279 w332]
      tunnel: [w289 w330] -> w242
      tunnel: [w288 w320] -> w233
      tunnel: [w287 w328] -> w241
      tunnel: [w286 w318] -> w240
      tunnel: [w285 w326] -> w239
      tunnel: [w284 w316] -> w238
      tunnel: [w283 w324] -> w237
      tunnel: [w282 w314] -> w236
      tunnel: [w281 w322] -> w235
      tunnel: [w280 w312] -> w234
      tunnel: w231 -> [w278 w311]
      tunnel: w230 -> [w277 w310]
      tunnel: w229 -> [w276 w309]
      tunnel: w228 -> [w275 w308]
      tunnel: w227 -> [w274 w307]
      tunnel: w226 -> [w273 w306]
      tunnel: [w272 w305] -> w218
      tunnel: [w271 w304] -> w217
      tunnel: [w269 w303] -> w216
      tunnel: [w270 w302] -> w215
      tunnel: [w268 w301] -> w214
      tunnel: [w267 w300] -> w213
      frame False {
        n157 = call "Step_Dir_to_CW_CCW.vi"("invert"=w279, "step"=w298, "direction"=w299) -> ("CCW"=w288:bool, "CW"=w289:bool)  [unwired: 7 in]
        n158 = call "Step_Dir_to_CW_CCW.vi"("invert"=w279, "step"=w296, "direction"=w297) -> ("CCW"=w286:bool, "CW"=w287:bool)  [unwired: 7 in]
        n159 = call "Step_Dir_to_CW_CCW.vi"("invert"=w279, "step"=w294, "direction"=w295) -> ("CCW"=w284:bool, "CW"=w285:bool)  [unwired: 7 in]
        n160 = call "Step_Dir_to_CW_CCW.vi"("invert"=w279, "step"=w292, "direction"=w293) -> ("CCW"=w282:bool, "CW"=w283:bool)  [unwired: 7 in]
        n161 = call "Step_Dir_to_CW_CCW.vi"("invert"=w279, "step"=w290, "direction"=w291) -> ("CCW"=w280:bool, "CW"=w281:bool)  [unwired: 7 in]
        n162 = call "Step_Dir_to_CW_CCW.vi"("invert"=w279, "step"=w277, "direction"=w278) -> ("CCW"=w271:bool, "CW"=w272:bool)  [unwired: 7 in]
        n163 = call "Step_Dir_to_CW_CCW.vi"("invert"=w279, "step"=w275, "direction"=w276) -> ("CCW"=w270:bool, "CW"=w269:bool)  [unwired: 7 in]
        n164 = call "Step_Dir_to_CW_CCW.vi"("invert"=w279, "step"=w273, "direction"=w274) -> ("CCW"=w267:bool, "CW"=w268:bool)  [unwired: 7 in]
      }
      frame True {
        n165 = case shown="False" w332 {
          tunnel: w331 -> [w348 w372]
          tunnel: [w348 w371] -> w330
          tunnel: w329 -> [w346 w370]
          tunnel: [w346 w369] -> w328
          tunnel: w327 -> [w344 w368]
          tunnel: [w344 w367] -> w326
          tunnel: w325 -> [w342 w366]
          tunnel: [w342 w365] -> w324
          tunnel: w323 -> [w340 w364]
          tunnel: [w340 w363] -> w322
          tunnel: w321 -> [w347 w362]
          tunnel: [w347 w362] -> w320
          tunnel: w319 -> [w345 w361]
          tunnel: [w345 w361] -> w318
          tunnel: w317 -> [w343 w360]
          tunnel: [w343 w360] -> w316
          tunnel: w315 -> [w341 w359]
          tunnel: [w341 w359] -> w314
          tunnel: w313 -> [w339 w358]
          tunnel: [w339 w358] -> w312
          tunnel: w311 -> [w338 w357]
          tunnel: w310 -> [w337 w350]
          tunnel: w309 -> [w336 w356]
          tunnel: w308 -> [w335 w352]
          tunnel: w307 -> [w334 w355]
          tunnel: w306 -> [w333 w353]
          tunnel: [w338 w349] -> w305
          tunnel: [w337 w350] -> w304
          tunnel: [w336 w351] -> w303
          tunnel: [w335 w352] -> w302
          tunnel: [w334 w354] -> w301
          tunnel: [w333 w353] -> w300
          frame False {
          }
          frame True {
            n166 = Not(x=w356) -> (.not. x?=w351:bool)
            n167 = Not(x=w355) -> (.not. x?=w354:bool)
            n168 = Not(x=w372) -> (.not. x?=w371:bool)
            n169 = Not(x=w370) -> (.not. x?=w369:bool)
            n170 = Not(x=w368) -> (.not. x?=w367:bool)
            n171 = Not(x=w366) -> (.not. x?=w365:bool)
            n172 = Not(x=w364) -> (.not. x?=w363:bool)
            n173 = Not(x=w357) -> (.not. x?=w349:bool)
          }
        }
      }
    }
    n174 = xnode "FPGA I/O Node"("Axis1_CW"=w242, "Axis1_CCW"=w233, "Axis2_CW"=w241, "Axis2_CCW"=w240, "Axis3_CW"=w239, "Axis3_CCW"=w238, "Axis4_CW"=w237, "Axis4_CCW"=w236, "Axis5_CW"=w235, "Axis5_CCW"=w234, "RMC/DIO10"=w218, "RMC/DIO11"=w217, "RMC/DIO12"=w216, "RMC/DIO13"=w215, "RMC/DIO15"=w214, "RMC/DIO17"=w213) -> ()  [unwired: 16 in, 16 out]
  }
  n175 = while {
    stop <- FALSE stop-if-true
    n176 = xnode "FPGA I/O Node"() -> ("RMC/DIO20"=w395:bool, "RMC/DIO21"=w394:bool, "RMC/DIO22"=w393:bool, "RMC/DIO23"=w392:bool, "RMC/DIO24"=w391:bool, "RMC/DIO25"=w390:bool, "RMC/DIO26"=w389:bool, "RMC/DIO27"=w388:bool)  [unwired: 8 in, 8 out]
    n177 = Build Array(w395, w394, w393, w392, w391, w390, w389, w388) -> (w376:bool[])
    n178 = Boolean Array To Number(Boolean array=w376) -> (number=→"DI (8bits)":u8)
    n179 = Number To Boolean Array(number="DO (8bits)") -> (Boolean array=w386:bool[])
    n180 = Index Array(array=w386) -> (element #1=w387:bool, element #2=w385:bool, element #3=w384:bool, element #4=w383:bool, element #5=w382:bool, element #6=w381:bool, element #7=w380:bool, element #8=w379:bool)  [unwired: 8 in]
    n181 = xnode "FPGA I/O Node"("RMC/DIO45"=w387, "RMC/DIO46"=w385, "RMC/DIO47"=w384, "RMC/DIO49"=w383, "RMC/DIO50"=w382, "RMC/DIO51"=w381, "RMC/DIO52"=w380, "RMC/DIO53"=w379) -> ()  [unwired: 8 in, 8 out]
  }
  n182 = timed-loop "Synchronization Loop" {
    timing: w6 -> [_]
    timing-out: [_] -> w5
    stop <- FALSE stop-if-true
    n183 = xnode "FPGA I/O Node"() -> ("Scan Clock"=w400:bool)  [unwired: 1 in, 1 out]
    n184 = global read "Global FPGA 8-axis.vi" "Sync Enable"() -> (w399:bool)
    n185 = Select(t="Sync Value", s="Sync Enable override?", f=w399) -> (s? t:f=w396:bool)
    n186 = call-poly <vilib>:"nism.scan.generateSyncScan.vi"("Scan Enable?"=w396, "Scan Clock"=w400) -> ("Timer Control"=w401:T6)  [unwired: 3 in]
    n187 = global write "Global FPGA 8-axis.vi" "Timer Control"(w401) -> ()
  }
  n188 = while {
    shift-right: [w407] -> _
    shift-left: FALSE ("RT Reset on Watchdog Failure?") -> [w406]
    stop <- FALSE stop-if-true
    # "Blink Loop"
    n189 = xnode "FPGA I/O Node"("FPGA LED"=w406) -> ()  [unwired: 1 in, 1 out]
    n190 = call "Wait"("Count(mSec)"=u8 100) -> ()  [unwired: 1 out]
    n191 = Not(x=w406) -> (.not. x?=w407:bool)
  }
  n192 = timed-loop "Reset Monitoring Loop" {
    timing: w4 -> [_]
    timing-out: [_] -> w3
    stop <- FALSE stop-if-true
    n193 = global read "Global FPGA 8-axis.vi" "Reset Pending"() -> (w411:bool[])
    n194 = xnode "FPGA I/O Node"() -> ("Scan Clock"=w410:bool)  [unwired: 1 in, 1 out]
    n195 = feedback-in #1(w410) -> ()
    n196 = feedback #1() -> (w409:bool)  [unwired: 1 in]
    n197 = Greater?(x=w410, y=w409) -> (0:w415:bool)
    n198 = feedback #2() -> (w414:bool[])  [unwired: 1 in]
    n199 = Select(t=w411, s=w415, f=w414) -> (s? t:f=w412:bool[])
    n200 = feedback-in #2(w412) -> ()
    n201 = global write "Global FPGA 8-axis.vi" "Reset"(w412) -> ()
  }
  n202 = node-c288(w3) -> ()
  n203 = node-c288(w5) -> ()
  n204 = node-c288(w7) -> ()
